vi "Globals.vi"() -> ()   [LabVIEW 2026]
panel:
  out "SavedFiles":path
  out "Fluid":u16=100
  out "GraphNbPoints":u16
  out "LastProcessFile":path
  out "task ID IO":u32 format="%.0x"
  out "LinearityFile":path
  out "Uspc":path
  out "Appli":path=path "c:/mhp-weld"
  out "Path COM":path=path "c:/mhp-weld/com.txt"
  in  "Mux Port RS (0..)":u8 caption="Host PC Port Com"
  in  "Host Port RS (0..)":u8 caption="SPS Port Com"
  out "ProcessParametersDir":path
  in  "PassWord":string="1234"
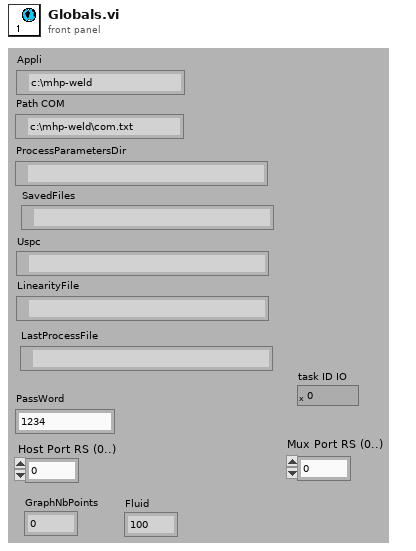
[diagram p1: front panel]
diagram:
